vi "Func-엑셀 데이터를 그래프로 출력.vi"() -> ()   [LabVIEW 2015] (continued)
1027.51\n1027.53\n1027.54\n1027.56\n1027.58\n1027.59\n1027.61\n1027.63\n1027.64\n1027.66\n1027.68\n1027.69\n1027.71\n1027.73\n1027.74\n1027.76\n1027.78\n1027.79\n1027.81\n1027.83\n1027.84\n1027.86\n1027.88\n1027.89\n1027.91\n1027.93\n1027.94\n1027.96\n1027.98\n1027.99\n1028.01\n1028.03\n1028.04\n1028.06\n1028.08\n1028.09\n1028.11\n1028.13\n1028.14\n1028.16\n1028.18\n1028.19\n1028.21\n1028.23\n1028.24\n1028.26\n1028.28\n1028.29\n1028.31\n1028.33\n1028.35\n1028.36\n1028.38\n1028.39\n1028.41\n1028.43\n1028.44\n1028.46\n1028.48\n1028.49\n1028.51\n1028.53\n1028.54\n1028.56\n1028.58\n1028.59\n1028.61\n1028.63\n1028.64\n1028.66\n1028.68\n1028.7\n1028.71\n1028.73\n1028.74\n1028.76\n1028.78\n1028.8\n1028.81\n1028.83\n1028.84\n1028.86\n1028.88\n1028.89\n1028.91\n1028.93\n1028.94\n1028.96\n1028.98\n1028.99\n1029.01\n1029.03\n1029.05\n1029.06\n1029.08\n1029.09\n1029.11\n1029.13\n1029.14\n1029.16\n1029.18\n1029.19\n1029.21\n1029.23\n1029.24\n1029.26\n1029.28\n1029.29\n1029.31\n1029.33\n1029.34\n1029.36\n1029.38\n1029.39\n1029.41\n1029.43\n1029.44\n1029.46\n1029.48\n1029.5\n1029.51\n1029.53\n1029.54\n1029.56\n1029.58\n1029.6\n1029.61\n1029.63\n1029.64\n1029.66\n1029.68\n1029.69\n1029.71\n1029.73\n1029.75\n1029.76\n1029.78\n1029.79\n1029.81\n1029.83\n1029.84\n1029.86\n1029.88\n1029.89\n1029.91\n1029.93\n1029.94\n1029.96\n1029.98\n1029.99\n1030.01\n1030.03\n1030.04\n1030.06\n1030.08\n1030.09\n1030.11\n1030.13\n1030.14\n1030.16\n1030.18\n1030.19\n1030.21\n1030.23\n1030.24\n1030.26\n1030.28\n1030.29\n1030.31\n1030.33\n1030.34\n1030.36\n1030.38\n1030.39\n1030.41\n1030.43\n1030.44\n1030.46\n1030.48\n1030.49\n1030.51\n1030.53\n1030.54\n1030.56\n1030.58\n1030.59\n1030.61\n1030.63\n1030.64\n1030.66\n1030.68\n1030.69\n1030.71\n1030.73\n1030.74\n1030.76\n1030.78\n1030.79\n1030.81\n1030.83\n1030.84\n1030.86\n1030.88\n1030.89\n1030.91\n1030.93\n1030.94\n1030.96\n1030.98\n1030.99\n1031.01\n1031.03\n1031.04\n1031.06\n1031.08\n1031.1\n1031.11\n1031.13\n1031.14\n1031.16\n1031.18\n1031.19\n1031.21\n1031.23\n1031.24\n1031.26\n1031.28\n1031.29\n1031.31\n1031.33\n1031.34\n1031.36\n1031.38\n1031.39\n1031.41\n1031.43\n1031.45\n1031.46\n1031.48\n1031.49\n1031.51\n1031.53\n1031.55\n1031.56\n1031.58\n1031.59\n1031.61\n1031.63\n1031.64\n1031.66\n1031.68\n1031.69\n1031.71\n1031.73\n1031.74\n1031.76\n1031.78\n1031.8\n1031.81\n1031.83\n1031.84\n1031.86\n1031.88\n1031.9\n1031.91\n1031.93\n1031.94\n1031.96\n1031.98\n1031.99\n1032.01\n1032.03\n1032.05\n1032.06\n1032.08\n1032.09\n1032.11\n1032.13\n1032.15\n1032.16\n1032.18\n1032.19\n1032.21\n1032.23\n1032.24\n1032.26\n1032.28\n1032.29\n1032.31\n1032.33\n1032.34\n1032.36\n1032.38\n1032.4\n1032.41\n1032.43\n1032.44\n1032.46\n1032.48\n1032.49\n1032.51\n1032.53\n1032.54\n1032.56\n1032.58\n1032.59\n1032.61\n1032.63\n1032.64\n1032.66\n1032.68\n1032.69\n1032.71\n1032.73\n1032.74\n1032.76\n1032.78\n1032.79\n1032.81\n1032.83\n1032.84\n1032.86\n1032.88\n1032.89\n1032.91\n1032.93\n1032.94\n1032.96\n1032.98\n1032.99\n1033.01\n1033.03\n1033.04\n1033.06\n1033.08\n1033.09\n1033.11\n1033.13\n1033.14\n1033.16\n1033.18\n1033.19\n1033.21\n1033.23\n1033.24\n1033.26\n1033.28\n1033.29\n1033.31\n1033.33\n1033.34\n1033.36\n1033.38\n1033.39\n1033.41\n1033.43\n1033.44\n1033.46\n1033.48\n1033.49\n1033.51\n1033.53\n1033.54\n1033.56\n1033.58\n1033.59\n1033.61\n1033.63\n1033.64\n1033.66\n1033.68\n1033.69\n1033.71\n1033.73\n1033.74\n1033.76\n1033.78\n1033.79\n1033.81\n1033.83\n1033.84\n1033.86\n1033.88\n1033.89\n1033.91\n1033.93\n1033.94\n1033.96\n1033.98\n1033.99\n1034.01\n1034.03\n1034.04\n1034.06\n1034.08\n1034.09\n1034.11\n1034.13\n1034.14\n1034.16\n1034.18\n1034.2\n1034.21\n1034.23\n1034.24\n1034.26\n1034.28\n1034.29\n1034.31\n1034.33\n1034.34\n1034.36\n1034.38\n1034.39\n1034.41\n1034.43\n1034.44\n1034.46\n1034.48\n1034.49\n1034.51\n1034.53\n1034.55\n1034.56\n1034.58\n1034.59\n1034.61\n1034.63\n1034.64\n1034.66\n1034.68\n1034.69\n1034.71\n1034.73\n1034.74\n1034.76\n1034.78\n1034.79\n1034.81\n1034.83\n1034.84\n1034.86\n1034.88\n1034.9\n1034.91\n1034.93\n1034.94\n1034.96\n1034.98\n1034.99\n1035.01\n1035.03\n1035.04\n1035.06\n1035.08\n1035.09\n1035.11\n1035.13\n1035.15\n1035.16\n1035.18\n1035.19\n1035.21\n1035.23\n1035.25\n1035.26\n1035.28\n1035.29\n1035.31\n1035.33\n1035.34\n1035.36\n1035.38\n1035.39\n1035.41\n1035.43\n1035.44\n1035.46\n1035.48\n1035.5\n1035.51\n1035.53\n1035.54\n1035.56\n1035.58\n1035.59\n1035.61\n1035.63\n1035.64\n1035.66\n1035.68\n1035.69\n1035.71\n1035.73\n1035.74\n1035.76\n1035.78\n1035.79\n1035.81\n1035.83\n1035.84\n1035.86\n1035.88\n1035.89\n1035.91\n1035.93\n1035.94\n1035.96\n1035.98\n1035.99\n1036.01\n1036.03\n1036.04\n1036.06\n1036.08\n1036.09\n1036.11\n1036.13\n1036.14\n1036.16\n1036.18\n1036.19\n1036.21\n1036.23\n1036.24\n1036.26\n1036.28\n1036.29\n1036.31\n1036.33\n1036.34\n1036.36\n1036.38\n1036.39\n1036.41\n1036.43\n1036.44\n1036.46\n1036.48\n1036.49\n1036.51\n1036.53\n1036.54\n1036.56\n1036.58\n1036.59\n1036.61\n1036.63\n1036.64\n1036.66\n1036.68\n1036.69\n1036.71\n1036.73\n1036.74\n1036.76\n1036.78\n1036.79\n1036.81\n1036.83\n1036.84\n1036.86\n1036.88\n1036.89\n1036.91\n1036.93\n1036.95\n1036.96\n1036.98\n1036.99\n1037.01\n1037.03\n1037.04\n1037.06\n1037.08\n1037.09\n1037.11\n1037.13\n1037.14\n1037.16\n1037.18\n1037.19\n1037.21\n1037.23\n1037.24\n1037.26\n1037.28\n1037.3\n1037.31\n1037.33\n1037.34\n1037.36\n1037.38\n1037.39\n1037.41\n1037.43\n1037.44\n1037.46\n1037.48\n1037.49\n1037.51\n1037.53\n1037.54\n1037.56\n1037.58\n1037.59\n1037.61\n1037.63\n1037.65\n1037.66\n1037.68\n1037.69\n1037.71\n1037.73\n1037.74\n1037.76\n1037.78\n1037.79\n1037.81\n1037.83\n1037.84\n1037.86\n1037.88\n1037.9\n1037.91\n1037.93\n1037.94\n1037.96\n1037.98\n1038\n1038.01\n1038.03\n1038.04\n1038.06\n1038.08\n1038.1\n1038.11\n1038.13\n1038.15\n1038.16\n1038.18\n1038.19\n1038.21\n1038.23\n1038.25\n1038.26\n1038.28\n1038.29\n1038.31\n1038.33\n1038.34\n1038.36\n1038.38\n1038.39\n1038.41\n1038.43\n1038.44\n1038.46\n1038.48\n1038.49\n1038.51\n1038.53\n1038.54\n1038.56\n1038.58\n1038.59\n1038.61\n1038.63\n1038.64\n1038.66\n1038.68\n1038.7\n1038.71\n1038.73\n1038.74\n1038.76\n1038.78\n1038.8\n1038.81\n1038.83\n1038.84\n1038.86\n1038.88\n1038.89\n1038.91\n1038.93\n1038.94\n1038.96\n1038.98\n1038.99\n1039.01\n1039.03\n1039.04\n1039.06\n1039.08\n1039.09\n1039.11\n1039.13\n1039.14\n1039.16\n1039.18\n1039.19\n1039.21\n1039.23\n1039.24\n1039.26\n1039.28\n1039.29\n1039.31\n1039.33\n1039.34\n1039.36\n1039.38\n1039.39\n1039.41\n1039.43\n1039.44\n1039.46\n1039.48\n1039.49\n1039.51\n1039.53\n1039.54\n1039.56\n1039.58\n1039.59\n1039.61\n1039.63\n1039.64\n1039.66\n1039.68\n1039.69\n1039.71\n1039.73\n1039.74\n1039.76\n1039.78\n1039.79\n1039.81\n1039.83\n1039.84\n1039.86\n1039.88\n1039.89\n1039.91\n1039.93\n1039.94\n1039.96\n1039.98\n1039.99\n1040.01\n1040.03\n1040.04\n1040.06\n1040.08\n1040.09\n1040.11\n1040.13\n1040.14\n1040.16\n1040.18\n1040.19\n1040.21\n1040.23\n1040.24\n1040.26\n1040.28\n1040.29\n1040.31\n1040.33\n1040.34\n1040.36\n1040.38\n1040.39\n1040.41\n1040.43\n1040.44\n1040.46\n1040.48\n1040.49\n1040.51\n1040.53\n1040.54\n1040.56\n1040.58\n1040.59\n1040.61\n1040.63\n1040.64\n1040.66\n1040.68\n1040.69\n1040.71\n1040.73\n1040.75\n1040.76\n1040.78\n1040.79\n1040.81\n1040.83\n1040.84\n1040.86\n1040.88\n1040.89\n1040.91\n1040.93\n1040.94\n1040.96\n1040.98\n1041\n1041.01\n1041.03\n1041.04\n1041.06\n1041.08\n1041.1\n1041.11\n1041.13\n1041.14\n1041.16\n1041.18\n1041.19\n1041.21\n1041.23\n1041.24\n1041.26\n1041.28\n1041.29\n1041.31\n1041.33\n1041.35\n1041.36\n1041.38\n1041.39\n1041.41\n1041.43\n1041.45\n1041.46\n1041.48\n1041.49\n1041.51\n1041.53\n1041.54\n1041.56\n1041.58\n1041.59\n1041.61\n1041.63\n1041.64\n1041.66\n1041.68\n1041.69\n1041.71\n1041.73\n1041.74\n1041.76\n1041.78\n1041.79\n1041.81\n1041.83\n1041.84\n1041.86\n1041.88\n1041.9\n1041.91\n1041.93\n1041.94\n1041.96\n1041.98\n1041.99\n1042.01\n1042.03\n1042.05\n1042.06\n1042.08\n1042.09\n1042.11\n1042.13\n1042.14\n1042.16\n1042.18\n1042.19\n1042.21\n1042.23\n1042.24\n1042.26\n1042.28\n1042.29\n1042.31\n1042.33\n1042.34\n1042.36\n1042.38\n1042.39\n1042.41\n1042.43\n1042.44\n1042.46\n1042.48\n1042.5\n1042.51\n1042.53\n1042.54\n1042.56\n1042.58\n1042.59\n1042.61\n1042.63\n1042.64\n1042.66\n1042.68\n1042.69\n1042.71\n1042.73\n1042.74\n1042.76\n1042.78\n1042.79\n1042.81\n1042.83\n1042.84\n1042.86\n1042.88\n1042.89\n1042.91\n1042.93\n1042.94\n1042.96\n1042.98\n1042.99\n1043.01\n1043.03\n1043.04\n1043.06\n1043.08\n1043.09\n1043.11\n1043.13\n1043.14\n1043.16\n1043.18\n1043.19\n1043.21\n1043.23\n1043.24\n1043.26\n1043.28\n1043.29\n1043.31\n1043.33\n1043.34\n1043.36\n1043.38\n1043.39\n1043.41\n1043.43\n1043.44\n1043.46\n1043.48\n1043.49\n1043.51\n1043.53\n1043.54\n1043.56\n1043.58\n1043.59\n1043.61\n1043.63\n1043.64\n1043.66\n1043.68\n1043.69\n1043.71\n1043.73\n1043.75\n1043.76\n1043.78\n1043.79\n1043.81\n1043.83\n1043.85\n1043.86\n1043.88\n1043.89\n1043.91\n1043.93\n1043.94\n1043.96\n1043.98\n1043.99\n1044.01\n1044.03\n1044.04\n1044.06\n1044.08\n1044.1\n1044.11\n1044.13\n1044.14\n1044.16\n1044.18\n1044.2\n1044.21\n1044.23\n1044.24\n1044.26\n1044.28\n1044.29\n1044.31\n1044.33\n1044.34\n1044.36\n1044.38\n1044.39\n1044.41\n1044.43\n1044.45\n1044.46\n1044.48\n1044.49\n1044.51\n1044.53\n1044.54\n1044.56\n1044.58\n1044.59\n1044.61\n1044.63\n1044.65\n1044.66\n1044.68\n1044.69\n1044.71\n1044.73\n1044.74\n1044.76\n1044.78\n1044.79\n1044.81\n1044.83\n1044.84\n1044.86\n1044.88\n1044.89\n1044.91\n1044.93\n1044.94\n1044.96\n1044.98\n1044.99\n1045.01\n1045.03\n1045.04\n1045.06\n1045.08\n1045.09\n1045.11\n1045.13\n1045.14\n1045.16\n1045.18\n1045.19\n1045.21\n1045.23\n1045.24\n1045.26\n1045.28\n1045.29\n1045.31\n1045.33\n1045.34\n1045.36\n1045.38\n1045.39\n1045.41\n1045.43\n1045.44\n1045.46\n1045.48\n1045.49\n1045.51\n1045.53\n1045.54\n1045.56\n1045.58\n1045.59\n1045.61\n1045.63\n1045.64\n1045.66\n1045.68\n1045.69\n1045.71\n1045.73\n1045.74\n1045.76\n1045.78\n1045.79\n1045.81\n1045.83\n1045.84\n1045.86\n1045.88\n1045.89\n1045.91\n1045.93\n1045.94\n1045.96\n1045.98\n1045.99\n1046.01\n1046.03\n1046.04\n1046.06\n1046.08\n1046.09\n1046.11\n1046.13\n1046.14\n1046.16\n1046.18\n1046.19\n1046.21\n1046.23\n1046.24\n1046.26\n1046.28\n1046.29\n1046.31\n1046.33\n1046.34\n1046.36\n1046.38\n1046.39\n1046.41\n1046.43\n1046.44\n1046.46\n1046.48\n1046.49\n1046.51\n1046.53\n1046.54\n1046.56\n1046.58\n1046.59\n1046.61\n1046.63\n1046.64\n1046.66\n1046.68\n1046.69\n1046.71\n1046.73\n1046.74\n1046.76\n1046.78\n1046.79\n1046.81\n1046.83\n1046.85\n1046.86\n1046.88\n1046.89\n1046.91\n1046.93\n1046.94\n1046.96\n1046.98\n1046.99\n1047.01\n1047.03\n1047.04\n1047.06\n1047.08\n1047.09\n1047.11\n1047.13\n1047.14\n1047.16\n1047.18\n1047.2\n1047.21\n1047.23\n1047.24\n1047.26\n1047.28\n1047.3\n1047.31\n1047.33\n1047.34\n1047.36\n1047.38\n1047.39\n1047.41\n1047.43\n1047.44\n1047.46\n1047.48\n1047.49\n1047.51\n1047.53\n1047.54\n1047.56\n1047.58\n1047.59\n1047.61\n1047.63\n1047.65\n1047.66\n1047.68\n1047.69\n1047.71\n1047.73\n1047.74\n1047.76\n1047.78\n1047.79\n1047.81\n1047.83\n1047.84\n1047.86\n1047.88\n1047.89\n1047.91\n1047.93\n1047.94\n1047.96\n1047.98\n1048\n1048.01\n1048.03\n1048.04\n1048.06\n1048.08\n1048.09\n1048.11\n1048.13\n1048.14\n1048.16\n1048.18\n1048.19\n1048.21\n1048.23\n1048.25\n1048.26\n1048.28\n1048.29\n1048.31\n1048.33\n1048.34\n1048.36\n1048.38\n1048.39\n1048.41\n1048.43\n1048.44\n1048.46\n1048.48\n1048.49\n1048.51\n1048.53\n1048.54\n1048.56\n1048.58\n1048.59\n1048.61\n1048.63\n1048.64\n1048.66\n1048.68\n1048.69\n1048.71\n1048.73\n1048.74\n1048.76\n1048.78\n1048.79\n1048.81\n1048.83\n1048.84\n1048.86\n1048.88\n1048.89\n1048.91\n1048.93\n1048.94\n1048.96\n1048.98\n1048.99\n1049.01\n1049.03\n1049.04\n1049.06\n1049.08\n1049.09\n1049.11\n1049.13\n1049.14\n1049.16\n1049.18\n1049.19\n1049.21\n1049.23\n1049.24\n1049.26\n1049.28\n1049.29\n1049.31\n1049.33\n1049.34\n1049.36\n1049.38\n1049.39\n1049.41\n1049.43\n1049.44\n1049.46\n1049.48\n1049.49\n1049.51\n1049.53\n1049.54\n1049.56\n1049.58\n1049.6\n1049.61\n1049.63\n1049.64\n1049.66\n1049.68\n1049.69\n1049.71\n1049.73\n1049.74\n1049.76\n1049.78\n1049.79\n1049.81\n1049.83\n1049.84\n1049.86\n1049.88\n1049.89\n1049.91\n1049.93\n1049.95\n1049.96\n1049.98\n1049.99\n1050.01\n1050.03\n1050.05\n1050.06\n1050.08\n1050.09\n1050.11\n1050.13\n1050.14\n1050.16\n1050.18\n1050.2\n1050.21\n1050.23\n1050.24\n1050.26\n1050.28\n1050.3\n1050.31\n1050.33\n1050.34\n1050.36\n1050.38\n1050.4\n1050.41\n1050.43\n1050.44\n1050.46\n1050.48\n1050.49\n1050.51\n1050.53\n1050.55\n1050.56\n1050.58\n1050.59\n1050.61\n1050.63\n1050.64\n1050.66\n1050.68\n1050.69\n1050.71\n1050.73\n1050.75\n1050.76\n1050.78\n1050.79\n1050.81\n1050.83\n1050.84\n1050.86\n1050.88\n1050.9\n1050.91\n1050.93\n1050.94\n1050.96\n1050.98\n1050.99\n1051.01\n1051.03\n1051.04\n1051.06\n1051.08\n1051.09\n1051.11\n1051.13\n1051.14\n1051.16\n1051.18\n1051.19\n1051.21\n1051.23\n1051.24\n1051.26\n1051.28\n1051.29\n1051.31\n1051.33\n1051.34\n1051.36\n1051.38\n1051.39\n1051.41\n1051.43\n1051.44\n1051.46\n1051.48\n1051.49\n1051.51\n1051.53\n1051.54\n1051.56\n1051.58\n1051.59\n1051.61\n1051.63\n1051.64\n1051.66\n1051.68\n1051.69\n1051.71\n1051.73\n1051.74\n1051.76\n1051.78\n1051.79\n1051.81\n1051.83\n1051.84\n1051.86\n1051.88\n1051.89\n1051.91\n1051.93\n1051.94\n1051.96\n1051.98\n1051.99\n1052.01\n1052.03\n1052.04\n1052.06\n1052.08\n1052.09\n1052.11\n1052.13\n1052.14\n1052.16\n1052.18\n1052.19\n1052.21\n1052.23\n1052.24\n1052.26\n1052.28\n1052.29\n1052.31\n1052.33\n1052.35\n1052.36\n1052.38\n1052.39\n1052.41\n1052.43\n1052.44\n1052.46\n1052.48\n1052.49\n1052.51\n1052.53\n1052.54\n1052.56\n1052.58\n1052.59\n1052.61\n1052.63\n1052.64\n1052.66\n1052.68\n1052.7\n1052.71\n1052.73\n1052.74\n1052.76\n1052.78\n1052.8\n1052.81\n1052.83\n1052.84\n1052.86\n1052.88\n1052.89\n1052.91\n1052.93\n1052.95\n1052.96\n1052.98\n1052.99\n1053.01\n1053.03\n1053.05\n1053.06\n1053.08\n1053.09\n1053.11\n1053.13\n1053.14\n1053.16\n1053.18\n1053.19\n1053.21\n1053.23\n1053.24\n1053.26\n1053.28\n1053.29\n1053.31\n1053.33\n1053.34\n1053.36\n1053.38\n1053.4\n1053.41\n1053.43\n1053.44\n1053.46\n1053.48\n1053.49\n1053.51\n1053.53\n1053.54\n1053.56\n1053.58\n1053.59\n1053.61\n1053.63\n1053.64\n1053.66\n1053.68\n1053.69\n1053.71\n1053.73\n1053.75\n1053.76\n1053.78\n1053.79\n1053.81\n1053.83\n1053.84\n1053.86\n1053.88\n1053.89\n1053.91\n1053.93\n1053.94\n1053.96\n1053.98\n1054\n1054.01\n1054.03\n1054.04\n1054.06\n1054.08\n1054.09\n1054.11\n1054.13\n1054.14\n1054.16\n1054.18\n1054.19\n1054.21\n1054.23\n1054.24\n1054.26\n1054.28\n1054.29\n1054.31\n1054.33\n1054.34\n1054.36\n1054.38\n1054.39\n1054.41\n1054.43\n1054.44\n1054.46\n1054.48\n1054.49\n1054.51\n1054.53\n1054.54\n1054.56\n1054.58\n1054.59\n1054.61\n1054.63\n1054.64\n1054.66\n1054.68\n1054.69\n1054.71\n1054.73\n1054.74\n1054.76\n1054.78\n1054.79\n1054.81\n1054.83\n1054.84\n1054.86\n1054.88\n1054.89\n1054.91\n1054.93\n1054.94\n1054.96\n1054.98\n1054.99\n1055.01\n1055.03\n1055.04\n1055.06\n1055.08\n1055.09\n1055.11\n1055.13\n1055.14\n1055.16\n1055.18\n1055.19\n1055.21\n1055.23\n1055.24\n1055.26\n1055.28\n1055.29\n1055.31\n1055.33\n1055.34\n1055.36\n1055.38\n1055.39\n1055.41\n1055.43\n1055.44\n1055.46\n1055.48\n1055.49\n1055.51\n1055.53\n1055.54\n1055.56\n1055.58\n1055.59\n1055.61\n1055.63\n1055.64\n1055.66\n1055.68\n1055.69\n1055.71\n1055.73\n1055.74\n1055.76\n1055.78\n1055.8\n1055.81\n1055.83\n1055.84\n1055.86\n1055.88\n1055.89\n1055.91\n1055.93\n1055.94\n1055.96\n1055.98\n1055.99\n1056.01\n1056.03\n1056.05\n1056.06\n1056.08\n1056.09\n1056.11\n1056.13\n1056.15\n1056.16\n1056.18\n1056.19\n1056.21\n1056.23\n1056.24\n1056.26\n1056.28\n1056.29\n1056.31\n1056.33\n1056.34\n1056.36\n1056.38\n1056.4\n1056.41\n1056.43\n1056.44\n1056.46\n1056.48\n1056.5\n1056.51\n1056.53\n1056.54\n1056.56\n1056.58\n1056.6\n1056.61\n1056.63\n1056.64\n1056.66\n1056.68\n1056.69\n1056.71\n1056.73\n1056.75\n1056.76\n1056.78\n1056.79\n1056.81\n1056.83\n1056.85\n1056.86\n1056.88\n1056.89\n1056.91\n1056.93\n1056.94\n1056.96\n1056.98\n1056.99\n1057.01\n1057.03\n1057.04\n1057.06\n1057.08\n1057.09\n1057.11\n1057.13\n1057.14\n1057.16\n1057.18\n1057.2\n1057.21\n1057.23\n1057.24\n1057.26\n1057.28\n1057.29\n1057.31\n1057.33\n1057.34\n1057.36\n1057.38\n1057.39\n1057.41\n1057.43\n1057.44\n1057.46\n1057.48\n1057.49\n1057.51\n1057.53\n1057.54\n1057.56\n1057.58\n1057.59\n1057.61\n1057.63\n1057.64\n1057.66\n1057.68\n1057.69\n1057.71\n1057.73\n1057.74\n1057.76\n1057.78\n1057.79\n1057.81\n1057.83\n1057.84\n1057.86\n1057.88\n1057.89\n1057.91\n1057.93\n1057.94\n1057.96\n1057.98\n1057.99\n1058.01\n1058.03\n1058.04\n1058.06\n1058.08\n1058.09\n1058.11\n1058.13\n1058.14\n1058.16\n1058.18\n1058.19\n1058.21\n1058.23\n1058.24\n1058.26\n1058.28\n1058.29\n1058.31\n1058.33\n1058.34\n1058.36\n1058.38\n1058.39\n1058.41\n1058.43\n1058.44\n1058.46\n1058.48\n1058.49\n1058.51\n1058.53\n1058.54\n1058.56\n1058.58\n1058.59\n1058.61\n1058.63\n1058.64\n1058.66\n1058.68\n1058.69\n1058.71\n1058.73\n1058.74\n1058.76\n1058.78\n1058.79\n1058.81\n1058.83\n1058.84\n1058.86\n1058.88\n1058.89\n1058.91\n1058.93\n1058.94\n1058.96\n1058.98\n1058.99\n1059.01\n1059.03\n1059.04\n1059.06\n1059.08\n1059.09\n1059.11\n1059.13\n1059.14\n1059.16\n1059.18\n1059.19\n1059.21\n1059.23\n1059.24\n1059.26\n1059.28\n1059.29\n1059.31\n1059.33\n1059.34\n1059.36\n1059.38\n1059.39\n1059.41\n1059.43\n1059.44\n1059.46\n1059.48\n1059.5\n1059.51\n1059.53\n1059.54\n1059.56\n1059.58\n1059.6\n1059.61\n1059.63\n1059.64\n1059.66\n1059.68\n1059.69\n1059.71\n1059.73\n1059.75\n1059.76\n1059.78\n1059.79\n1059.81\n1059.83\n1059.85\n1059.86\n1059.88\n1059.89\n1059.91\n1059.93\n1059.95\n1059.96\n1059.98\n1059.99\n1060.01\n1060.03\n1060.05\n1060.06\n1060.08\n1060.1\n1060.11\n1060.13\n1060.14\n1060.16\n1060.18\n1060.19\n1060.21\n1060.23\n1060.24\n1060.26\n1060.28\n1060.29\n1060.31\n1060.33\n1060.34\n1060.36\n1060.38\n1060.39\n1060.41\n1060.43\n1060.45\n1060.46\n1060.48\n1060.49\n1060.51\n1060.53\n1060.54\n1060.56\n1060.58\n1060.59\n1060.61\n1060.63\n1060.64\n1060.66\n1060.68\n1060.69\n1060.71\n1060.73\n1060.74\n1060.76\n1060.78\n1060.79\n1060.81\n1060.83\n1060.84\n1060.86\n1060.88\n1060.89\n1060.91\n1060.93\n1060.94\n1060.96\n1060.98\n1060.99\n1061.01\n1061.03\n1061.04\n1061.06\n1061.08\n1061.09\n1061.11\n1061.13\n1061.14\n1061.16\n1061.18\n1061.19\n1061.21\n1061.23\n1061.24\n1061.26\n1061.28\n1061.29\n1061.31\n1061.33\n1061.34\n1061.36\n1061.38\n1061.39\n1061.41\n1061.43\n1061.44\n1061.46\n1061.48\n1061.49\n1061.51\n1061.53\n1061.54\n1061.56\n1061.58\n1061.59\n1061.61\n1061.63\n1061.64\n1061.66\n1061.68\n1061.69\n1061.71\n1061.73\n1061.74\n1061.76\n1061.78\n1061.79\n1061.81\n1061.83\n1061.84\n1061.86\n1061.88\n1061.9\n1061.91\n1061.93\n1061.94\n1061.96\n1061.98\n1061.99\n1062.01\n1062.03\n1062.04\n1062.06\n1062.08\n1062.09\n1062.11\n1062.13\n1062.14\n1062.16\n1062.18\n1062.19\n1062.21\n1062.23\n1062.25\n1062.26\n1062.28\n1062.29\n1062.31\n1062.33\n1062.35\n1062.36\n1062.38\n1062.39\n1062.41\n1062.43\n1062.44\n1062.46\n1062.48\n1062.49\n1062.51\n1062.53\n1062.54\n1062.56\n1062.58\n1062.6\n1062.61\n1062.63\n1062.64\n1062.66\n1062.68\n1062.7\n1062.71\n1062.73\n1062.74\n1062.76\n1062.78\n1062.79\n1062.81\n1062.83\n1062.84\n1062.86\n1062.88\n1062.89\n1062.91\n1062.93\n1062.95\n1062.96\n1062.98\n1062.99\n1063.01\n1063.03\n1063.04\n1063.06\n1063.08\n1063.09\n1063.11\n1063.13\n1063.14\n1063.16\n1063.18\n1063.2\n1063.21\n1063.23\n1063.24\n1080.57\n1080.74\n1080.91\n1081.08\n1081.25\n1081.41\n1081.58\n1081.75\n1081.91\n1082.08\n1082.25\n1082.41\n1082.58\n1082.75\n1082.91\n1083.08\n1083.26\n1083.42\n1083.59\n1083.76\n1083.92\n1084.09\n1084.26\n1084.42\n1084.59\n1084.76\n1084.93\n1085.1\n1085.27\n1085.44\n1085.61\n1085.77\n1085.95\n1086.11\n1086.28\n1086.46\n1086.62\n1086.79\n1086.96\n1087.12\n1087.29\n1087.46\n1087.63\n1087.8\n1087.96\n1088.13\n1088.3\n1088.46\n1088.63\n1088.81\n1088.97\n1089.14\n1089.31\n1089.47\n1089.64\n1089.81\n1089.97\n1090.14\n1090.31\n1090.47\n1090.64\n1090.81\n1090.97\n1091.14\n1091.31\n1091.47\n1091.64\n1091.81\n1091.97\n1092.14\n1092.31\n1092.47\n1092.64\n1092.81\n1092.97\n1093.14\n1093.31\n1093.47\n1093.64\n1093.81\n1093.97\n1094.15\n1094.32
